vi "case_demo.vi"() -> ()   [LabVIEW 2017]
panel:
  in  "Enum":enum16{""}(ring)
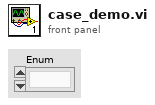
[diagram p1: front panel]
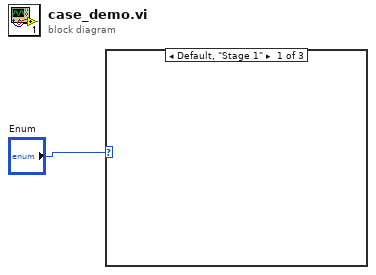
[diagram p0: block diagram]
diagram:
  n1 = case shown="Default, \"Stage 1\"" "Enum" {
    frame 2, Default {
    }
    frame "" {
    }
    frame 1 {
    }
  }
